vi "Set_TestMode.vi"(8 "error in (no error)":errorcluster) -> (0 "error out":errorcluster)   [LabVIEW 2019]
uses:
  Set_config/cmd_setPara.ctl
  Glob_setting.vi
panel:
  out "6.3.9 시험시간":dbl format="%#_g 시간"
  out "6.3.8 시험시간":dbl format="%#_g 시간"
  out "6.3.6 시험시간":dbl format="%#_g 시간"
  out "6.3.4 시험시간":dbl format="%#_g 시간"
  out "6.3.3 시험시간":dbl format="%#_g 시간"
  out "6.3.2 시험시간":dbl format="%#_g 시간"
  in  "6.3.9 사이클":dbl
  in  "6.3.8 사이클":dbl
  in  "6.3.6 사이클":dbl
  in  "6.3.4 사이클":dbl
  in  "6.3.3 사이클":dbl
  in  "6.3.2 사이클":dbl
  in  "Apply":bool
  in  "6.3.9 OFF":dbl
  in  "6.3.9 ON":dbl
  in  "6.3.9 시간":dbl
  in  "6.3.8 작동":dbl
  in  "6.3.8 시간":dbl
  in  "6.3.6 작동 2":dbl
  in  "6.3.6 미작동":dbl
  in  "6.3.6 작동 1":dbl
  in  "6.3.4 미작동":dbl
  in  "6.3.4 작동":dbl
  in  "6.3.3 미작동":dbl
  in  "6.3.3 작동":dbl
  in  "6.3.2 미작동":dbl
  in  "6.3.2 작동":dbl
  in  "Exit":bool
  # "ES 규격 시험 절차"
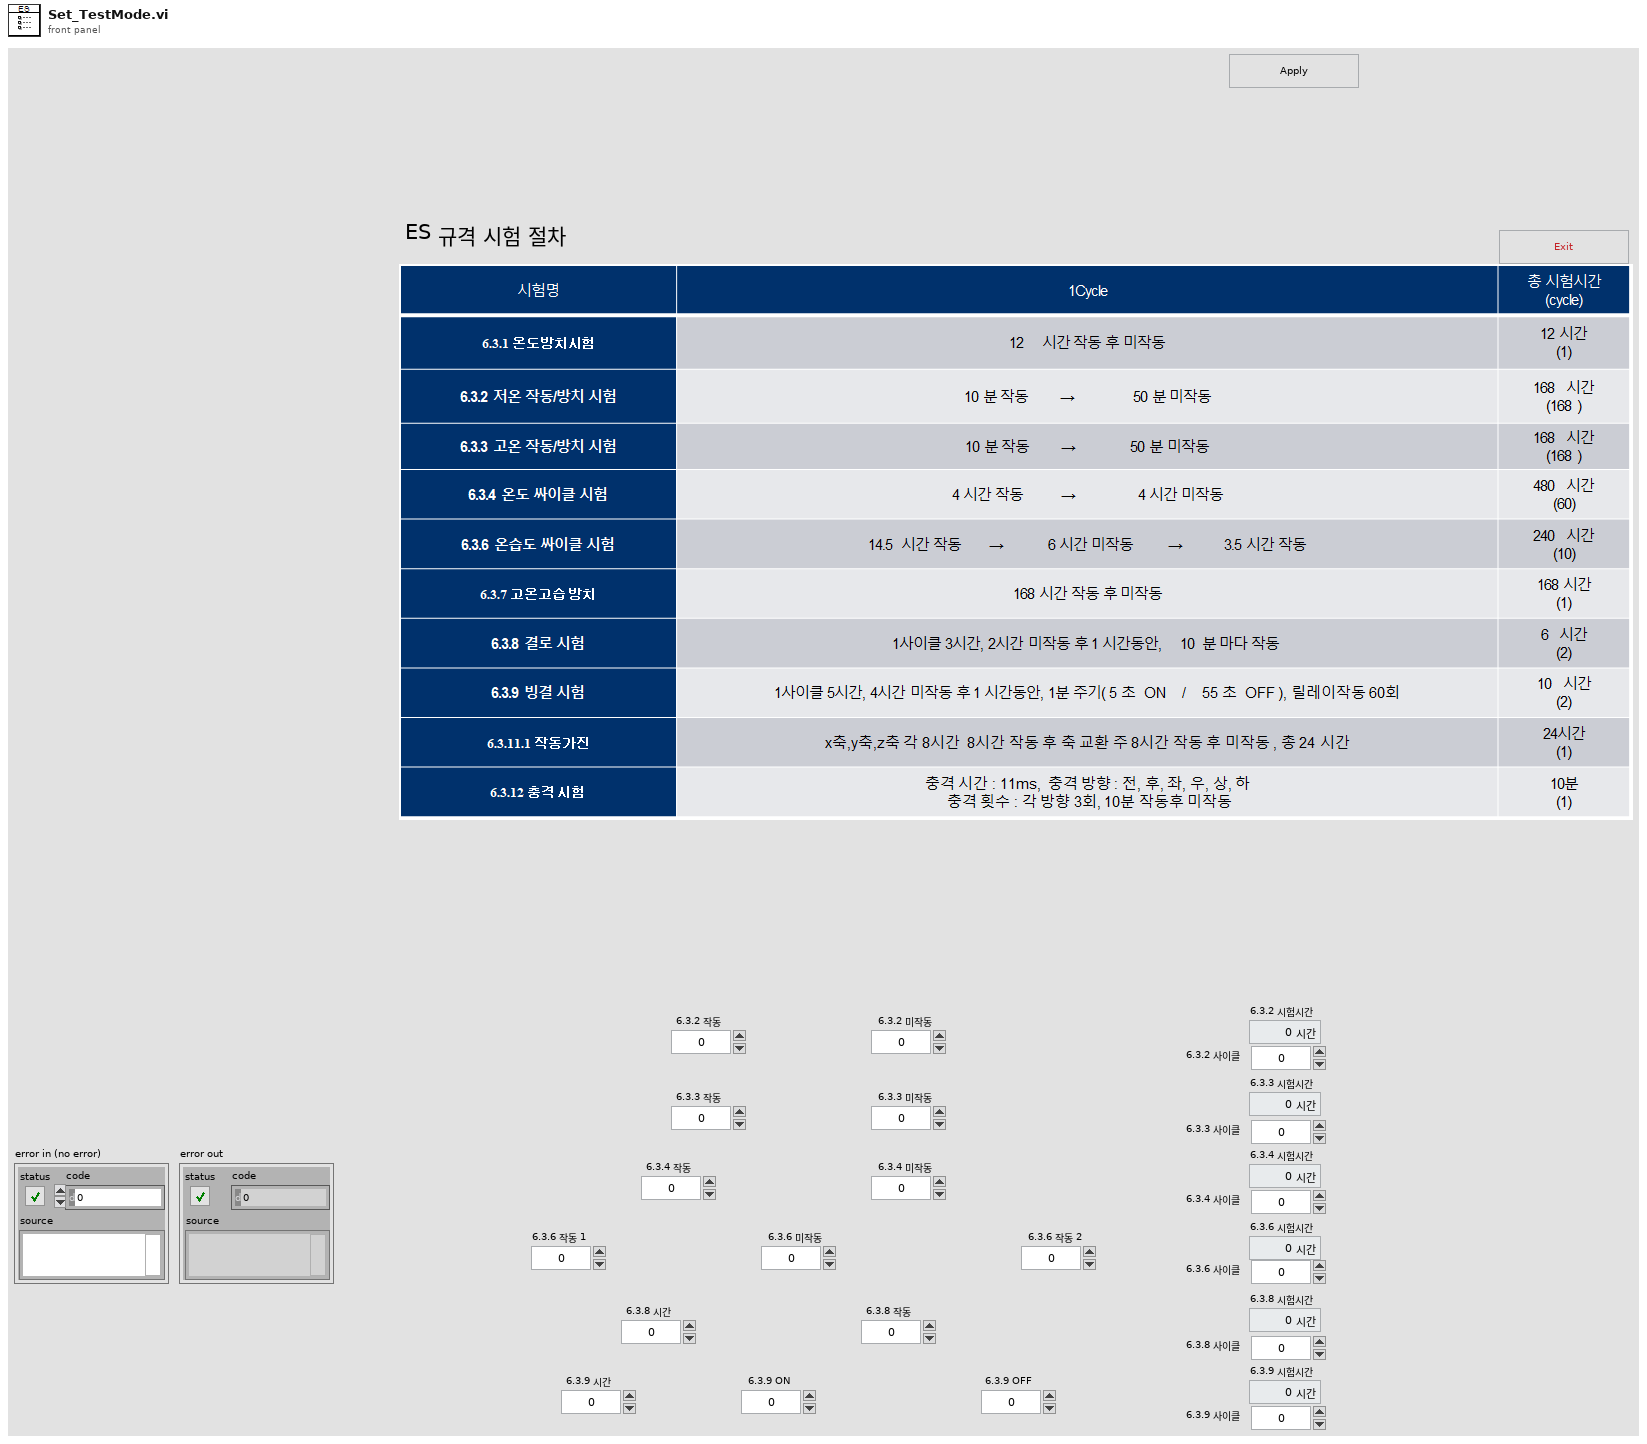
[diagram p1: front panel]
types:
  T1 = typedef "cmd_setPara.ctl" = enum16{"init", "write", "read", "default"}
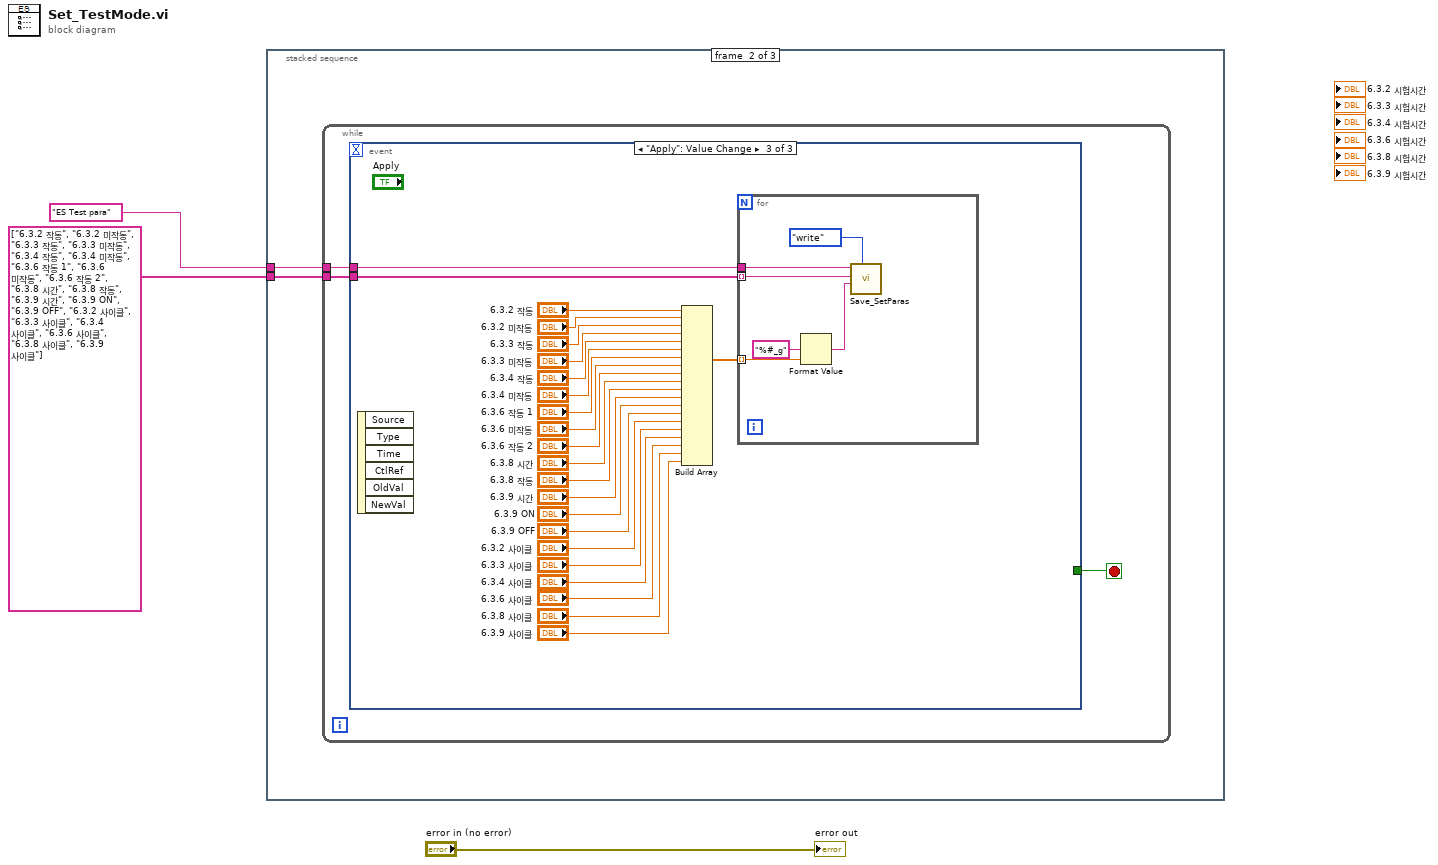
[diagram p0: block diagram]
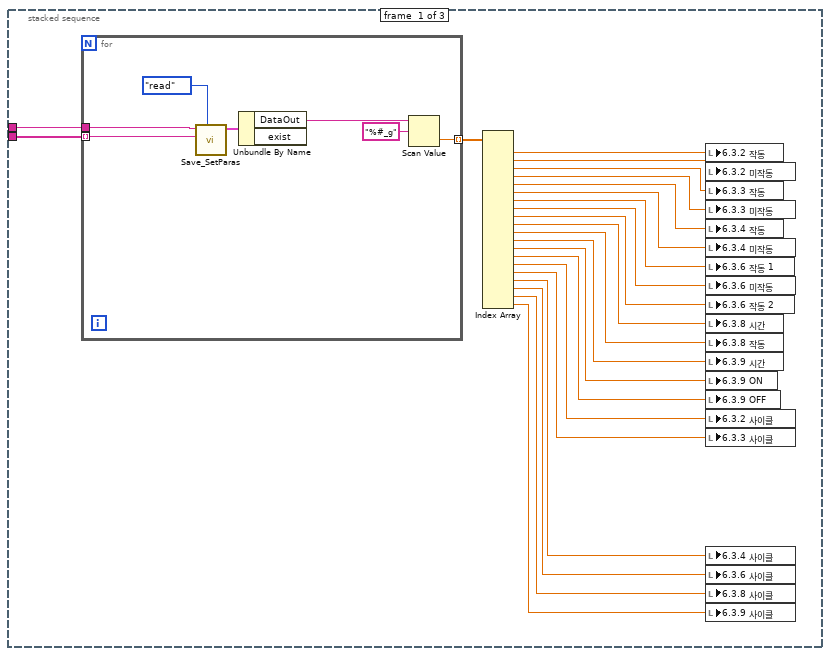
[diagram p2: hidden frame]
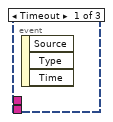
[diagram p3: hidden frame]
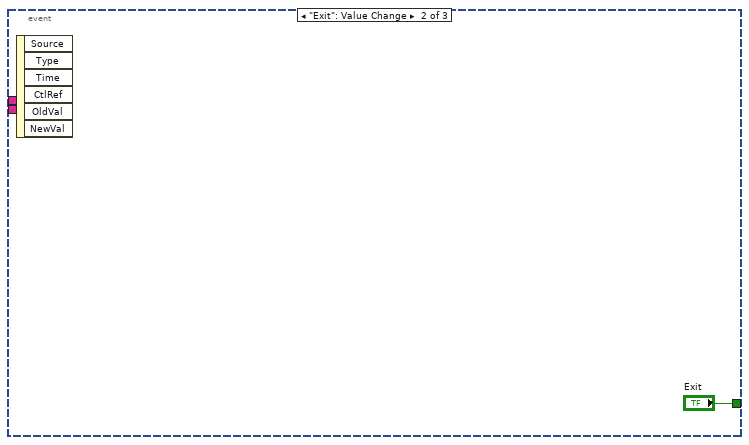
[diagram p4: hidden frame]
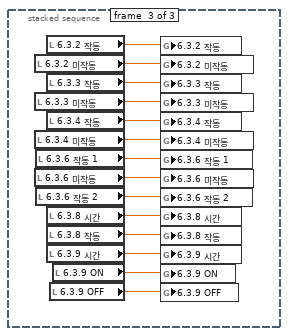
[diagram p5: hidden frame]
diagram:
  n1 = stacked-sequence {
    tunnel: "ES Test para" -> [w26 w35 _]
    tunnel: string[] ["6.3.2 작동", "6.3.2 미작동", "6.3.3 작동", "6.3.3 미작동", "6.3.4 작동", "6.3.4 미작동", "6.3.6 작동 1", "6.3.6 미작동", "6.3.6 작동 2", "6.3.8 시간", "6.3.8 작동", "6.3.9 시간", "6.3.9 ON", "6.3.9 OFF", "6.3.2 사이클", "6.3.3 사이클", "6.3.4 사이클", "6.3.6 사이클", "6.3.8 사이클", "6.3.9 사이클"] -> [w25 w34 _]
    frame #0 {
      n2 = for {
        tunnel: w25 -> [w32] mode=indexing
        tunnel: w26 -> [w30]
        tunnel: [w27] -> w24 mode=indexing
        n3 = call "Save_SetParas.vi"("cmd"=cmd_setPara."read", "Key"=w32, "Section"=w30) -> ("dataout"=w31:cluster{"DataOut":string, "exist":bool})  [unwired: 7 in, 1 out]
        n4 = Unbundle By Name(w31) -> ("DataOut"=w29:string)  [unwired: 1 out]
        n5 = Scan Value(string=w29, format string="%#_g") -> (value=w27:dbl)  [unwired: 1 in, 1 out]
      }
      n6 = Index Array(array=w24) -> (element #1=w23:dbl, element #2=w22:dbl, element #3=w21:dbl, element #4=w20:dbl, element #5=w19:dbl, element #6=w18:dbl, element #7=w17:dbl, element #8=w16:dbl, element #9=w15:dbl, element #10=w14:dbl, element #11=w13:dbl, element #12=w12:dbl, element #13=w11:dbl, element #14=w10:dbl, element #15=w9:dbl, element #16=w8:dbl, element #17=w7:dbl, element #18=w6:dbl, element #19=w5:dbl, element #20=w4:dbl)  [unwired: 20 in]
      n7 = local write "6.3.2 작동"(w23) -> ()
      n8 = local write "6.3.2 미작동"(w22) -> ()
      n9 = local write "6.3.3 작동"(w21) -> ()
      n10 = local write "6.3.3 미작동"(w20) -> ()
      n11 = local write "6.3.4 작동"(w19) -> ()
      n12 = local write "6.3.4 미작동"(w18) -> ()
      n13 = local write "6.3.6 작동 1"(w17) -> ()
      n14 = local write "6.3.6 미작동"(w16) -> ()
      n15 = local write "6.3.6 작동 2"(w15) -> ()
      n16 = local write "6.3.8 시간"(w14) -> ()
      n17 = local write "6.3.8 작동"(w13) -> ()
      n18 = local write "6.3.9 시간"(w12) -> ()
      n19 = local write "6.3.9 ON"(w11) -> ()
      n20 = local write "6.3.9 OFF"(w10) -> ()
      n21 = local write "6.3.2 사이클"(w9) -> ()
      n22 = local write "6.3.3 사이클"(w8) -> ()
      n23 = local write "6.3.4 사이클"(w7) -> ()
      n24 = local write "6.3.6 사이클"(w6) -> ()
      n25 = local write "6.3.8 사이클"(w5) -> ()
      n26 = local write "6.3.9 사이클"(w4) -> ()
    }
    frame #1 {
      n27 = while {
        tunnel: w35 -> [w37]
        tunnel: w34 -> [w36]
        stop <- w38 stop-if-true
        n28 = event shown="[2] \"Apply\": Value Change" {
          selector: _ -> [_ _ _]
          dyn-events: _ -> [_ _ _]
          timeout: _ -> [_ _ _]
          tunnel: [_ "Exit" _] -> w38
          tunnel: w37 -> [_ _ w62]
          tunnel: w36 -> [_ _ w61]
          event Timeout {
            n29 = event-data() -> ()  [unwired: 1 in, 3 out]
          }
          event "Exit": Value Change {
            n30 = event-data() -> ()  [unwired: 1 in, 6 out]
          }
          event "Apply": Value Change {
            n31 = event-data() -> ()  [unwired: 1 in, 6 out]
            n32 = Build Array("6.3.2 작동", "6.3.2 미작동", "6.3.3 작동", "6.3.3 미작동", "6.3.4 작동", "6.3.4 미작동", "6.3.6 작동 1", "6.3.6 미작동", "6.3.6 작동 2", "6.3.8 시간", "6.3.8 작동", "6.3.9 시간", "6.3.9 ON", "6.3.9 OFF", "6.3.2 사이클", "6.3.3 사이클", "6.3.4 사이클", "6.3.6 사이클", "6.3.8 사이클", "6.3.9 사이클") -> (w46:dbl[])
            n33 = for {
              tunnel: w62 -> [w68]
              tunnel: w61 -> [w67] mode=indexing
              tunnel: w46 -> [w66] mode=indexing
              n34 = Format Value(format string="%#_g", value (0)=w66) -> (output string=w65:string)  [unwired: 1 in]
              n35 = call "Save_SetParas.vi"("cmd"=cmd_setPara."write", "Data"=w65, "Key"=w67, "Section"=w68) -> ()  [unwired: 6 in, 2 out]
            }
          }
        }
      }
    }
    frame #2 {
      n36 = local read "6.3.2 미작동"() -> (w81:dbl)
      n37 = local read "6.3.3 미작동"() -> (w79:dbl)
      n38 = local read "6.3.4 미작동"() -> (w77:dbl)
      n39 = local read "6.3.6 미작동"() -> (w75:dbl)
      n40 = local read "6.3.6 작동 1"() -> (w76:dbl)
      n41 = local read "6.3.6 작동 2"() -> (w74:dbl)
      n42 = local read "6.3.2 작동"() -> (w82:dbl)
      n43 = local read "6.3.3 작동"() -> (w80:dbl)
      n44 = local read "6.3.4 작동"() -> (w78:dbl)
      n45 = local read "6.3.8 시간"() -> (w73:dbl)
      n46 = local read "6.3.8 작동"() -> (w72:dbl)
      n47 = local read "6.3.9 시간"() -> (w71:dbl)
      n48 = local read "6.3.9 OFF"() -> (w69:dbl)
      n49 = local read "6.3.9 ON"() -> (w70:dbl)
      n50 = global write "Glob_setting.vi" "6.3.2 작동"(w82) -> ()
      n51 = global write "Glob_setting.vi" "6.3.2 미작동"(w81) -> ()
      n52 = global write "Glob_setting.vi" "6.3.3 작동"(w80) -> ()
      n53 = global write "Glob_setting.vi" "6.3.3 미작동"(w79) -> ()
      n54 = global write "Glob_setting.vi" "6.3.4 작동"(w78) -> ()
      n55 = global write "Glob_setting.vi" "6.3.4 미작동"(w77) -> ()
      n56 = global write "Glob_setting.vi" "6.3.6 작동 1"(w76) -> ()
      n57 = global write "Glob_setting.vi" "6.3.6 미작동"(w75) -> ()
      n58 = global write "Glob_setting.vi" "6.3.6 작동 2"(w74) -> ()
      n59 = global write "Glob_setting.vi" "6.3.8 시간"(w73) -> ()
      n60 = global write "Glob_setting.vi" "6.3.8 작동"(w72) -> ()
      n61 = global write "Glob_setting.vi" "6.3.9 시간"(w71) -> ()
      n62 = global write "Glob_setting.vi" "6.3.9 ON"(w70) -> ()
      n63 = global write "Glob_setting.vi" "6.3.9 OFF"(w69) -> ()
    }
  }
  "error out" <- "error in (no error)"
